vi "Main.vi"() -> ()   [LabVIEW 2013] (continued)
                n3557 = case shown="1" w6177 {
                  tunnel: w6176 -> [w6190 _]
                  frame 1 {
                    # "2nd Data Point.\nUpdate Status of c: an u: in cRIO"
                    n3558 = Index Array(array=w6190) -> (element #1=w6189:bool, element #2=w6186:bool)  [unwired: 2 in]
                    n3559 = Select(t="c: OK,", s=w6189, f="c: Fail,") -> (s? t:f=w6182:string)
                    n3560 = Select(t=" u: OK.", s=w6186, f=" u: Fail.") -> (s? t:f=w6181:string)
                    n3561 = Concatenate Strings("{Running Process} cRIO data file created status: ", w6182, w6181) -> (w6179:string)
                    n3562 = call "Queue - EnQueue to MessageQ.vi"("<NoD> Don't Display to UI"=TRUE, "Message"=w6179) -> ()  [unwired: 9 in, 1 out]
                  }
                  frame 0, Default {
                    # "Skip 1st Data Point"
                  }
                }
                n3563 = Increment(x=w6177) -> (x+1=w6178:i32)
              }
            }
          }
        }
        "Samples/ch Count" <- w5678
        n3564 = case shown="True" w5666 {
          tunnel: w5664 -> [w5698 w5745]
          tunnel: w5676 -> [w5702 w5774]
          tunnel: [w5702 w5772] -> w5675
          tunnel: [_ w5767] -> w5665
          tunnel: [w5701 w5756] -> w5673
          tunnel: w5672 -> [w5701 w5770]
          tunnel: [_ w5763] -> w5667
          tunnel: w5661 -> [_ w5750]
          frame False {
            # "t-t0"
            # "Time Not Elapse"
            n3565 = local read "Key Values"() -> (w5700:T10)
            n3566 = Bundle By Name(cluster=w5700, "Recording Duration"=w5698) -> (w5699:T10)
            n3567 = local write "Key Values"(w5699) -> ()
            n3568 = Wait Until Next ms Multiple(millisecond multiple=u32 100) -> ()  [unwired: 1 out]
            n3569 = feedback #1(0) -> (w5696:i32)
            n3570 = case shown="0" w5696 {
              frame 1, Default {
              }
              frame 0 {
                # "0 - no change"
                # "Every 10 Counts = 1sec"
                n3571 = local read "% Hold Flashing FLAG"() -> (w5707:bool)
                n3572 = Not(x=w5707) -> (.not. x?=→"% Hold Flashing FLAG":bool)
                n3573 = case shown="True" w5707 {
                  tunnel: [w5715 w5727] -> w5708
                  tunnel: 3.0 ("lower limit") -> [w5710 w5722]
                  tunnel: [u32 0 w5721] -> w5703
                  tunnel: u32 655580 -> [_ w5720]
                  frame False {
                    # "Minus When False"
                    n3574 = local read "% Hold. Time Completed"() -> (w5711:dbl)
                    n3575 = In Range and Coerce(upper limit=95.0, x=w5711, lower limit=10.0) -> (In Range?=w5712:bool)  [unwired: 1 out]
                    n3576 = case shown="False" w5712 {
                      tunnel: [w5716 w5719] -> w5715
                      tunnel: w5711 -> [w5716 w5718]
                      tunnel: w5710 -> [_ w5717]
                      frame False {
                      }
                      frame True {
                        n3577 = Subtract(x=w5718, y=w5717) -> (x-y=w5719:dbl)
                      }
                    }
                  }
                  frame True {
                    # "Add when TRUE"
                    n3578 = local read "% Hold. Time Completed"() -> (w5724:dbl)
                    n3579 = In Range and Coerce(upper limit=90.0, x=w5724, lower limit=5.0) -> (In Range?=w5723:bool)  [unwired: 1 out]
                    n3580 = case shown="True" w5723 {
                      tunnel: [w5729 w5733] -> w5727
                      tunnel: w5724 -> [w5729 w5732]
                      tunnel: w5722 -> [_ w5731]
                      tunnel: [u32 0 w5730] -> w5721
                      tunnel: w5720 -> [_ w5730]
                      frame False {
                      }
                      frame True {
                        n3581 = Add(x=w5732, y=w5731) -> (x+y=w5733:dbl)
                      }
                    }
                  }
                }
                n3582 = local write "% Hold. Time Completed"(w5708) -> ()
                n3583 = disable-structure shown="Disabled" {
                  frame Disabled {
                    # "We will not write the numerical\nindicator here :)"
                    n3584 = local read "% Hold. Time Completed (Num)"() -> ()  [unwired: 1 in]
                  }
                  frame Enabled {
                  }
                }
                n3585 = property class="DigNum (strict)"("NumText.FontColor"=w5703) -> ()  [unwired: 2 in, 2 out]
              }
            }
            n3586 = Increment(x=w5696) -> (x+1=w5694:i32)
            n3587 = Quotient & Remainder(x=w5694, y=10) -> (x-y*floor(x/y)=w5692:i32)  [unwired: 1 out]
            n3588 = feedback-in #1(w5692) -> ()
          }
          frame True {
            # "ProgStatus\n1 - Not running (Background)\n2 - RUN (Green)\n4 - RUN HLD (Red)\n8 - HLD Flashing (Red)"
            # "Segment.Type\n0 - End\n1 - Rate\n3 - Dwell"
            # "ProgStatus\n1 - Not running\n2 - RUN\n4 - RUN HLD\n8 - HLD Flashing"
            # "Time Elapsed"
            n3589 = local read "VISA resource name RS232"() -> (w5769:string)
            n3590 = local read "Simulate ET3500"() -> (w5735:bool)
            n3591 = local read "ET3500 Error"() -> (w5768:errorcluster)
            n3592 = control-ref of="ET3504 Status"() -> (w5743:refnum<vi>)
            n3593 = call "ET3500 - Read Program Parameters.vi"("Sample/ch per Count"=w5750, "Simulate"=w5735, "ET3500 Status"=w5743, "error in (no error)"=w5768, "subVI (Auto Interactive)"=TRUE ("subVI"), "Option"=cluster{"Init":bool, "Close":bool} {"Init"=FALSE, "Close"=FALSE}, "VISA resource name"=w5769) -> ("error out"=w5759:errorcluster, "Segment.Type"=w5758:i16, "Parameter Cluster (Scaled)"=w5757:T76, "Segment.Duration (min)"=w5771:dbl)  [unwired: 1 out]
            "Parameter Cluster (Scaled)" <- w5757
            n3594 = local read "TransactionRunNo (Execute)"() -> (w5752:string)
            n3595 = Unbundle By Name(w5757) -> ("SegTimeLeft (min)"=w5776:dbl, "PVIn (degC)"=w5741:dbl, "ProgStatus"=w5775:i16)
            n3596 = local read "Transaction No (Execute)"() -> (w5754:string)
            n3597 = control-ref of="WPS Details Setup"() -> (w5755:refnum<vi>)
            n3598 = control-ref of="Sequence Status"() -> (w5760:refnum<vi>)
            n3599 = control-ref of="MCListBox FHS Setup"() -> (w5761:refnum<vi>)
            n3600 = And(x=w5735, y="Simulate Hold Temp Inc") -> (x .and. y?=w5739:bool)
            n3601 = local read "DB - Active Process"() -> (w5744:bool)
            n3602 = local read "DB - Transaction"() -> (w5751:bool)
            n3603 = Bundle("Transaction No (Execute)"=w5754, "TransactionRunNo (Execute)"=w5752) -> (w5753:T77)  [unwired: 1 in]
            n3604 = Select(t="Simulate Hold Temp Inc", s=w5739, f=0.0) -> (s? t:f=w5737:dbl)
            n3605 = Select(t=errorcluster {"status"=TRUE, "code"=-1000, "source"="Simulate ET3500 Error. "} ("Error Out"), s="Simulate ET3500 Error", f=w5759) -> (s? t:f=w5763:errorcluster)
            n3606 = Add(x=w5741, y=w5737) -> (x+y=w5740:dbl)
            n3607 = call "Status - Update Sequence Status.vi"("Sequence Status"=w5760, "WPS Details"=w5755, "DB - Transaction"=w5751, "Transaction"=w5753, "MCListBox FHS Setup"=w5761, "ET3504 Status"=w5743, "Error In"=w5759, "Parameter Cluster (Scaled)"=w5757, "DB - Active Process"=w5744, "Segment.Type"=w5758) -> ("Segment.Type II"=w5756:i16, "Error Out"=→"System Status":errorcluster)  [unwired: 4 in]
            n3608 = local write "ET3500 Error"(w5763) -> ()
            n3609 = To Long Integer(number=w5775) -> (32bit integer=w5773:i32)
            n3610 = case shown="\"Running\"" w5774 {
              selector: w5774 -> [w5798 w5807 w5830]
              tunnel: w5773 -> [w5802 w5810 _]
              tunnel: [w5799 w5808 w5830] -> w5772
              tunnel: [_ _ TRUE] -> w5767
              tunnel: w5740 -> [_ w5806 _]
              frame "Wait For RUN", Default {
                n3611 = Equal?(x=w5802, y=2) -> (x = y?=w5800:bool)
                n3612 = case shown="True" w5800 {
                  tunnel: [w5803 ET3500_Program_Status."Running"] -> w5799
                  tunnel: w5798 -> [w5803 _]
                  frame False {
                  }
                  frame True {
                  }
                }
              }
              frame "Running" {
                # "Wait For Stop"
                n3613 = case shown="True" "Stop On Final Target Temperature" {
                  tunnel: w5810 -> [w5813 _]
                  tunnel: [w5811 w5824] -> w5809
                  tunnel: w5806 -> [_ w5816]
                  frame False {
                    n3614 = Equal?(x=w5813, y=1) -> (x = y?=w5811:bool)
                  }
                  frame True {
                    # "If error any of these\nwill be  ZERO.\nThis is now the ERROR\ncheck condition\nof this STATE"
                    n3615 = local read "Final Target Temperature"() -> (w5823:cluster{"Final Target Temperature":string})
                    n3616 = Unbundle By Name(w5823) -> ("Final Target Temperature"=w5822:string)
                    n3617 = local read "Hold Time Completed"() -> (w5825:bool)
                    n3618 = local read "1st TC"() -> (w5817:dbl)
                    n3619 = Decimal String To Number(string=w5822) -> (number=w5820:i32)  [unwired: 2 in, 1 out]
                    n3620 = Add(x="Final Target Temp Offset", y=w5820) -> (x+y=w5819:i32)
                    "Final Target + Offset\n(Updated Only when active)" <- w5819
                    n3621 = Less Or Equal?(x=w5817, y=w5819) -> (x <= y?=w5818:bool)
                    n3622 = Less Or Equal?(x=w5816, y=w5819) -> (x <= y?=w5826:bool)
                    n3623 = Multiply(x=w5817, y=w5816) -> (x*y=w5815:dbl)
                    n3624 = Greater Than 0?(x=w5815) -> (x > 0?=w5814:bool)
                    n3625 = Compound Arithmetic op=AND "AND"(w5814, w5818, w5826, w5825) -> (w5824:bool)
                  }
                }
                n3626 = case shown="False" w5809 {
                  tunnel: [w5827 ET3500_Program_Status."Stopped"] -> w5808
                  tunnel: w5807 -> [w5827 _]
                  frame False {
                    # "Keep Waiting"
                  }
                  frame True {
                    # "Stopped"
                  }
                }
              }
              frame "Stopped" {
              }
            }
            n3627 = case shown="3" w5756 {
              tunnel: [w5836 w5927 w6039] -> w5742
              tunnel: w5776 -> [_ w5929 _]
              tunnel: w5771 -> [_ w5938 _]
              tunnel: w5770 -> [w5832 w5941 _]
              tunnel: w5740 -> [w5831 w5931 _]
              frame 0, Default {
                # "Not Ended yet?"
                # "CURRENT STATE:   End (0) or Rate (1) or ERROR"
                n3628 = case shown="3" w5832 {
                  tunnel: w5831 -> [_ w5867]
                  frame 0, Default {
                    # "PREVIOUS STATE:   End (0) or ERROR"
                  }
                  frame 3 {
                    w5853 = 1  # Value
                    w5852 = 2  # Recorded Hold Time
                    w5865 = cluster{"Color Box":u32, "Color Box 2":u32}[] [{"Color Box"=16711680, "Color Box 2"=16711680}, {"Color Box"=6618880, "Color Box 2"=6618880}, {"Color Box"=4934475, "Color Box 2"=4934475}, {"Color Box"=6618880, "Color Box 2"=6618880}]  # False is Now RED (Prev Grey)
                    # "PREVIOUS STATE:  Dwell (3)\nSo now Main Hold (Dwell) is OVER"
                    n3629 = local read "DB - Transaction"() -> (w5862:bool)
                    n3630 = local read "Simulate cRIO"() -> (w5848:bool)
                    n3631 = local read "Simulated TimeStamp"() -> (w5849:timestamp)
                    n3632 = local read "Parameter (Start Dwell Time)"() -> (w5864:timestamp)
                    n3633 = Get Date/Time In Seconds() -> (seconds since 1Jan1904=w5861:timestamp)
                    n3634 = And(x="Simulate Hold Time Inc", y=w5848) -> (x .and. y?=w5846:bool)
                    n3635 = Select(t="Simulate Hold Time Inc (s)", s=w5846, f=0.0) -> (s? t:f=w5843:dbl)
                    n3636 = Add(x=w5849, y=w5843) -> (x+y=w5842:timestamp)
                    n3637 = Select(t=w5842, s=w5848, f=w5861) -> (s? t:f=w5860:timestamp)
                    "Parameter (End Dwell Time)" <- w5860
                    n3638 = local read "Display Start Stop Marker"() -> (w5854:bool)
                    n3639 = local read "Info."() -> (w5863:T9)
                    n3640 = call "Parameters - Update.vi"("Parameter (End Dwell Temp)"=w5867, "Parameter (End Dwell Time)"=w5860, "Parameter (Start Dwell Time)"=w5864, "Info."=w5863) -> ("Variant Allowed (Hold Time)"=w5841:bool, "Cluster"=w5866:T78, "Parameters"=w5851:string[][])  [unwired: 4 in, 1 out]
                    n3641 = property on="Variant Allowed (Hold Time)" class="Bool (strict)"("Colors [4]"=w5865, "Value"=w5841) -> ()  [unwired: 2 in, 2 out]
                    n3642 = Index Array(array=w5851, index (row)=w5852, index (col)=w5853) -> (element=w5850:string)
                    n3643 = case shown="False" w5841 {
                      tunnel: w5850 -> [w5874 w5877]
                      frame True {
                        # "Hold Duration Variant OK."
                        n3644 = Concatenate Strings("{RUNNING Process} " ("string"), "Recorded Hold Duration is " ("string"), w5874, " (HH:MM)" ("string")) -> (w5872:string)
                        n3645 = call "Queue - EnQueue to MessageQ.vi"("<NoD> Don't Display to UI"=TRUE, "Message"=w5872) -> ()  [unwired: 9 in, 1 out]
                      }
                      frame False {
                        # "Hold Duration Variant Failed!"
                        n3646 = flat-sequence {
                          tunnel: w5877 -> [w5879]
                          tunnel: ["<E 306>"] -> w5876
                          frame #0 {
                            n3647 = Format Date/Time String() -> ()  [unwired: 3 in, 1 out]
                            "<current hold time> ON Failing Hold Time Variance" <- w5879
                          }
                        }
                        n3648 = property on="Toggle ET3500 Error" class="Str"("Val(Sgnl)"=w5876) -> ()  [unwired: 2 in, 2 out]
                      }
                    }
                    n3649 = case shown="True" w5854 {
                      tunnel: w5860 -> [_ w5881]
                      frame False {
                      }
                      frame True {
                        n3650 = To Double Precision Float(number=w5881) -> (double precision float=w5883:dbl)
                        n3651 = property on="Chart" class="WFChart (strict)"() -> ("XScale.MarkerVals[]"=w5880:dbl[])  [unwired: 2 in, 2 out]
                        n3652 = Build Array (concatenate)(w5880, w5883) -> (w5882:dbl[])
                        n3653 = property on="Chart" class="WFChart (strict)"("XScale.MarkerVals[]"=w5882) -> ()  [unwired: 2 in, 2 out]
                      }
                    }
                    n3654 = Unbundle By Name(w5866) -> ("End Holding Time & Date"=w5857:string, "End Holding Temperature"=w5856:string)
                    n3655 = property on="End Holding Time and Date" class="Str"("Value"=w5857) -> (error out=w5859:errorcluster)  [unwired: 2 in, 1 out]
                    n3656 = property on="End Holding Temperature" class="Str"("Value"=w5856) -> (error out=w5858:errorcluster)  [unwired: 2 in, 1 out]
                    n3657 = case shown="True" w5841 {
                      frame False {
                      }
                      frame True {
                        n3658 = property on="% Hold. Time Completed" class="Slide (strict)"() -> ("Scale.Maximum"=w5868:dbl)  [unwired: 2 in, 2 out]
                        n3659 = local write "% Hold. Time Completed (Num)"(w5868) -> ()
                        n3660 = local write "% Hold. Time Completed"(w5868) -> ()
                        n3661 = local write "Hold Time Completed"(TRUE ("Hold Time Completed")) -> ()
                      }
                    }
                    n3662 = Merge Errors(w5859, w5858) -> (w5855:errorcluster)
                    n3663 = case shown="True" w5862 {
                      tunnel: w5851 -> [_ w5917]
                      tunnel: w5857 -> [_ w5906]
                      tunnel: w5856 -> [_ w5916]
                      tunnel: w5841 -> [_ w5897]
                      tunnel: w5855 -> [w5884 _]
                      frame False {
                        n3664 = local read "Latest stp file"() -> (w5890:path)
                        n3665 = control-ref of="Parameter Buffer"() -> (w5891:refnum<vi>)
                        n3666 = call <vilib>:"Open Config Data.vi"("error in (no error)"=w5884, "create file if necessary (T)"=FALSE, "configuration file path"=w5890) -> ("error out"=w5887:errorcluster, "refnum"=w5889:T59)  [unwired: 6 in, 1 out]
                        n3667 = call "Key - Cluster Write.vi"("error in (no error)"=w5887, "Cluster Ref in"=w5891, "Refnum in"=w5889) -> ("error out"=w5886:errorcluster, "Refnum out"=w5888:T59)  [unwired: 7 in]
                        n3668 = call <vilib>:"Close Config Data.vi"("error in (no error)"=w5886, "write file if changed (T)"=TRUE, "refnum"=w5888) -> ("error out"=w5892:errorcluster)  [unwired: 7 in, 1 out]
                        n3669 = local write "stp file Error Out"(w5892) -> ()
                      }
                      frame True {
                        w5911 = T63[] [enum."[EndHoldTime]", enum."[HoldTimePercentage]", enum."[HoldProgressColor]"] items=["[IsActive]", "[TransactionNo]", "[TransactionRunNo]", "[SequenceStatus]", "[StartRecordTime]", "[EndRecordTime]", "[StartHoldTime]", "[EndHoldTime]", "[Message1]", "[Message2]", "[HoldTimeRemaining]", "[HoldTimePercentage]", "[HoldProgressColor]", "[OrderNumbers]", "[CurrentTemp]", "[UnitOfTemperature]", "[IsAppClientLive]", "[RawDataFile]", "[RecordedMinutes]", "[FurnaceControlStatus]", "[FurnaceControlColor]", "[ControllerStatus]", "[ControllerColor]", "[IsControllerOnline]", "[ProcessColor]", "[OverallColor]", "[LastUpdatedOn]", "[LastUpdatedCmsTime]", "[Inactive]"] ("[Execute].[ActiveProcess]\n2014-10-14 14:58")
                        w5912 = 2  # Recorded Hold Time
                        w5925 = T62[] [enum."[EndHoldTime]", enum."[EndHoldTemp]", enum."[HoldDurationMinutes]", enum."[HoldTimePercentage]", enum."[IsTimeWithinTol]"] items=["[StartRecordTime]", "[StartRecordTemp]", "[MaxRecordedTemp]", "[MaxRecordedTempTime]", "[MinRecordedTemp]", "[MinRecordedTempTime]", "[EndRecordTemp]", "[EndRecordTime]", "[RecordedMinutes]", "[StartHoldTime]", "[StartHoldTemp]", "[HoldTimeMaxTemp]", "[HoldTimeMaxTempTime]", "[HoldTimeMinTemp]", "[HoldTimeMinTempTime]", "[EndHoldTime]", "[EndHoldTemp]", "[HoldDurationMinutes]", "[TempDiffDuringHold]", "[UnitOfTemperature]", "[PerformedBy]", "[PerformedOn]", "[IsTempWithinTol]", "[IsTimeWithinTol]", "[HoldTimePercentage]", "[ProcessStatus]", "[OverallStatus]", "[SequenceStatus]", "[Parameter1]", "[Parameter2]", "[Parameter3]", "[Parameter4]", "[Parameter5]", "[Parameter6]", "[Parameter7]", "[Parameter8]", "[Parameter9]", "[Parameter10]", "[Parameter11]", "[Parameter12]", "[Result]", "[RawDataFile]", "[RawDataFilePath]", "[RawDataFileName]", "[OutputSetId]", "[SavedBy]", "[SavedOn]", "[Inactive]"]  # [TransactionResult] v02
                        # "[TempDiffDuringHold] will be updated when Recipe End ONLY"
                        n3670 = local read "Hold Time %"() -> (w5895:string)
                        n3671 = Select(t="1", s=w5897, f="0") -> (s? t:f=w5910:string)
                        n3672 = Select(t="100", s=w5897, f=w5895) -> (s? t:f=w5894:string)
                        n3673 = Index Array(array=w5917, index (col)=1 ("disabled index (col)")) -> (element=w5914:string[])  [unwired: 1 in]
                        n3674 = Index Array(array=w5914, index=w5912) -> (element=w5913:string)
                        n3675 = local read "TransactionRunNo"() -> (w5919:string)
                        n3676 = local read "Transaction No"() -> (w5920:string)
                        n3677 = Bundle("Transaction No"=w5920, "TransactionRunNo"=w5919) -> (w5918:T61)  [unwired: 1 in]
                        n3678 = Build Array(w5906, w5916, w5913, w5894, w5910) -> (w5924:string[])
                        n3679 = call "DB - [Execute].[Transaction].vi"("DB.Schema.Table"="SRTRS.Execute.TransactionResult", "Transaction"=w5918, "DB - Execute Transaction"=DB_-_Execute_Transaction_Enum."UPDATE [TransactionResult]" ("DB - Setup Item Enum"), "[TransactionResult] v02"=w5925, "<Values>"=w5924) -> ("SUMMARY"=w5902:errorcluster)  [unwired: 11 in, 3 out]
                        n3680 = local write "DB"(w5902) -> ()
                        n3681 = control-ref of="Hold Time Completed"() -> (w5900:refnum<vi>)
                        n3682 = global read "Global SRTRS.vi" "Logon"() -> (w5909:T21)
                        n3683 = Unbundle By Name(w5909) -> ("PlantID"=w5908:string, "SystemID"=w5907:string)
                        n3684 = call "String - Boolean Ref Color.vi"("Bool Refnum"=w5900) -> ("Color (U32 String)"=w5899:string)  [unwired: 4 in]
                        n3685 = Bundle("PlantID"=w5908, "SystemID"=w5907) -> (w5901:cluster{"PlantID":string, "SystemID":string})  [unwired: 1 in]
                        n3686 = Build Array(w5906, w5894, w5899) -> (w5905:string[])
                        n3687 = call "DB - [CMS].[Execute].[ActiveProcess].vi"("Application"="SRTRS", "[PlantId],[SystemId]"=w5901, "DB - CMS Execute ActiveProcess"=T74."UPDATE [Execute].[ActiveProcess]" ("DB - Execute ActiveProcess"), "[Execute].[ActiveProcess]\n2014-10-14 14:58"=w5911, "<Data>"=w5905) -> ("SUMMARY"=w5903:errorcluster)  [unwired: 11 in, 3 out]
                        n3688 = local write "DB"(w5903) -> ()
                      }
                    }
                  }
                }
                n3689 = local read "Parameter (End Dwell Time)"() -> (w5835:timestamp)
                n3690 = Equal?(x=w5835, y=timestamp(3471350400 s since 1904-01-01)) -> (x = y?=w5833:bool)
                n3691 = case shown="False" w5833 {
                  tunnel: [0.0 ("(HH:mm)") w5838] -> w5836
                  frame False {
                    # "Started and Ended"
                  }
                  frame True {
                    # "Not Started Yet"
                    n3692 = local read "Info."() -> (w5840:T9)
                    n3693 = Unbundle By Name(w5840) -> ("Hold. Time (hour:minute)"=w5839:string)
                    n3694 = call "String - Format to (HH_colon_MM).vi"("xx:xx"=w5839) -> ("seconds"=w5838:dbl)  [unwired: 9 in, 1 out]
                  }
                }
              }
              frame 3 {
                # "Hold Time (seconds)"
                # "CURRENT STATE:   Dwell (3) - Main Hold"
                n3695 = Divide(x=w5929, y=w5938) -> (x/y=w5933:dbl)
                n3696 = Subtract(x=1.0, y=w5933) -> (x-y=w5932:dbl)
                n3697 = Multiply(x=100.0, y=w5932) -> (x*y=w5930:dbl)
                n3698 = case shown="3, Default" w5941 {
                  tunnel: w5931 -> [w5942 w6003]
                  tunnel: w5930 -> [w5948 _]
                  frame 3, Default {
                    # "If FALSE previously, it will remain FALSE"
                    # "PREVIOUS STATE: Dwelling OR ERROR"
                    n3699 = local read "DB - Transaction"() -> (w5952:bool)
                    n3700 = local read "Info."() -> (w5953:T9)
                    n3701 = call "Parameters - Update.vi"("Parameter (Current Dwell Temp)"=w5942, "Info."=w5953) -> ("Variant Allowed (Current Hold Temp)"=w5944:bool)  [unwired: 6 in, 3 out]
                    n3702 = property on="Variant Allowed (Hold Temp)" class="Bool (strict)"() -> ("Value"=w5945:bool)  [unwired: 2 in, 2 out]
                    n3703 = And(x=w5945, y=w5944) -> (x .and. y?=w5946:bool)
                    n3704 = Number To Decimal String(number=w5948) -> (decimal integer string=w5947:string)  [unwired: 1 in]
                    "Hold Time %" <- w5947
                    n3705 = case shown="True" w5952 {
                      tunnel: w5946 -> [_ w5981]
                      tunnel: w5947 -> [_ w5972]
                      frame False {
                      }
                      frame True {
                        w5983 = T62[] [enum."[IsTempWithinTol]", enum."[HoldTimePercentage]"] items=["[StartRecordTime]", "[StartRecordTemp]", "[MaxRecordedTemp]", "[MaxRecordedTempTime]", "[MinRecordedTemp]", "[MinRecordedTempTime]", "[EndRecordTemp]", "[EndRecordTime]", "[RecordedMinutes]", "[StartHoldTime]", "[StartHoldTemp]", "[HoldTimeMaxTemp]", "[HoldTimeMaxTempTime]", "[HoldTimeMinTemp]", "[HoldTimeMinTempTime]", "[EndHoldTime]", "[EndHoldTemp]", "[HoldDurationMinutes]", "[TempDiffDuringHold]", "[UnitOfTemperature]", "[PerformedBy]", "[PerformedOn]", "[IsTempWithinTol]", "[IsTimeWithinTol]", "[HoldTimePercentage]", "[ProcessStatus]", "[OverallStatus]", "[SequenceStatus]", "[Parameter1]", "[Parameter2]", "[Parameter3]", "[Parameter4]", "[Parameter5]", "[Parameter6]", "[Parameter7]", "[Parameter8]", "[Parameter9]", "[Parameter10]", "[Parameter11]", "[Parameter12]", "[Result]", "[RawDataFile]", "[RawDataFilePath]", "[RawDataFileName]", "[OutputSetId]", "[SavedBy]", "[SavedOn]", "[Inactive]"]  # [TransactionResult] 2014-09-28 19:20
                        # "The indicator can show 25:59:59\ni.e. more than 23:59:59"
                        n3706 = Select(t="1", s=w5981, f="0") -> (s? t:f=w5978:string)
                        n3707 = local read "TransactionRunNo"() -> (w5975:string)
                        n3708 = Build Array(w5978, w5972) -> (w5982:string[])
                        n3709 = local read "Transaction No"() -> (w5976:string)
                        n3710 = Bundle("Transaction No"=w5976, "TransactionRunNo"=w5975) -> (w5974:T61)  [unwired: 1 in]
                        n3711 = call "DB - [Execute].[Transaction].vi"("DB.Schema.Table"="SRTRS.Execute.TransactionResult", "Transaction"=w5974, "DB - Execute Transaction"=DB_-_Execute_Transaction_Enum."UPDATE [TransactionResult]" ("DB - Setup Item Enum"), "[TransactionResult] v02"=w5983, "<Values>"=w5982) -> ("SUMMARY"=w5973:errorcluster)  [unwired: 11 in, 3 out]
                        n3712 = local write "DB"(w5973) -> ()
                      }
                    }
                    n3713 = Compound Arithmetic op=AND(w5945, invert w5944) -> (w5943:bool)
                    n3714 = property on="Variant Allowed (Hold Temp)" class="Bool (strict)"("Value"=w5946) -> ()  [unwired: 2 in, 2 out]
                    n3715 = case shown="True" w5943 {
                      tunnel: w5942 -> [_ w5955]
                      frame False {
                      }
                      frame True {
                        # "1st Time Variant Failed!"
                        n3716 = flat-sequence {
                          tunnel: w5955 -> [w5959]
                          tunnel: ["<E 305>" ("Value (Signaling)")] -> w5954
                          frame #0 {
                            n3717 = Number To Fractional String(number=w5959, precision (6)=i16 0) -> (F-format string=→"<current temperature> ON Failing Hold Temp Variance":string)  [unwired: 2 in]
                          }
                        }
                        n3718 = property on="Toggle ET3500 Error" class="Str"("Val(Sgnl)"=w5954) -> ()  [unwired: 2 in, 2 out]
                      }
                    }
                    n3719 = local read "Enable Central Monitoring"() -> (w5950:bool)
                    n3720 = local read "DB - Active Process"() -> (w5951:bool)
                    n3721 = And(x=w5950, y=w5951) -> (x .and. y?=w5949:bool)
                    n3722 = case shown="True" w5949 {
                      tunnel: w5947 -> [_ w5964]
                      frame False {
                      }
                      frame True {
                        w5967 = T63[] [enum."[HoldTimePercentage]", enum."[HoldProgressColor]"] items=["[IsActive]", "[TransactionNo]", "[TransactionRunNo]", "[SequenceStatus]", "[StartRecordTime]", "[EndRecordTime]", "[StartHoldTime]", "[EndHoldTime]", "[Message1]", "[Message2]", "[HoldTimeRemaining]", "[HoldTimePercentage]", "[HoldProgressColor]", "[OrderNumbers]", "[CurrentTemp]", "[UnitOfTemperature]", "[IsAppClientLive]", "[RawDataFile]", "[RecordedMinutes]", "[FurnaceControlStatus]", "[FurnaceControlColor]", "[ControllerStatus]", "[ControllerColor]", "[IsControllerOnline]", "[ProcessColor]", "[OverallColor]", "[LastUpdatedOn]", "[LastUpdatedCmsTime]", "[Inactive]"] ("[Execute].[ActiveProcess]\n2014-10-14 14:58")
                        n3723 = global read "Global SRTRS.vi" "Logon"() -> (w5970:T21)
                        n3724 = control-ref of="Hold Time Completed"() -> (w5962:refnum<vi>)
                        n3725 = Unbundle By Name(w5970) -> ("PlantID"=w5969:string, "SystemID"=w5968:string)
                        n3726 = call "String - Boolean Ref Color.vi"("Bool Refnum"=w5962) -> ("Color (U32 String)"=w5961:string)  [unwired: 4 in]
                        n3727 = Bundle("PlantID"=w5969, "SystemID"=w5968) -> (w5963:cluster{"PlantID":string, "SystemID":string})  [unwired: 1 in]
                        n3728 = Build Array(w5964, w5961) -> (w5966:string[])
                        n3729 = call "DB - [CMS].[Execute].[ActiveProcess].vi"("Application"="SRTRS", "[PlantId],[SystemId]"=w5963, "DB - CMS Execute ActiveProcess"=T74."UPDATE [Execute].[ActiveProcess]" ("DB - Execute ActiveProcess"), "[Execute].[ActiveProcess]\n2014-10-14 14:58"=w5967, "<Data>"=w5966) -> ("SUMMARY"=w5965:errorcluster)  [unwired: 11 in, 3 out]
                        n3730 = local write "DB"(w5965) -> ()
                      }
                    }
                  }
                  frame 1, 300 {
                    w6001 = cluster{"Color Box":u32, "Color Box 2":u32}[] [{"Color Box"=16711680, "Color Box 2"=16711680}, {"Color Box"=6618880, "Color Box 2"=6618880}, {"Color Box"=4934475, "Color Box 2"=4934475}, {"Color Box"=6618880, "Color Box 2"=6618880}]  # False is Now RED, (Prev  Grey)
                    w5991 = cluster{"Color Box":u32, "Color Box 2":u32}[] [{"Color Box"=16383786, "Color Box 2"=16383786}, {"Color Box"=6618880, "Color Box 2"=6618880}, {"Color Box"=4934475, "Color Box 2"=4934475}, {"Color Box"=6618880, "Color Box 2"=6618880}]  # False is Now Yellow (Prev Grey)
                    # "Create Start Hold Marker"
                    # "Fix ERROR here"
                    # "Initialized to TRUE"
                    # "PREVIOUS STATE:  Rate (1) or Dwell (300) => Just Entering Dwell (3)"
                    n3731 = local read "DB - Transaction"() -> (w5999:bool)
                    n3732 = local read "Simulated TimeStamp"() -> (w5998:timestamp)
                    n3733 = local read "Simulate cRIO"() -> (w5996:bool)
                    n3734 = Get Date/Time In Seconds() -> (seconds since 1Jan1904=w5997:timestamp)
                    n3735 = Select(t=w5998, s=w5996, f=w5997) -> (s? t:f=w5995:timestamp)
                    "Parameter (Start Dwell Time)" <- w5995
                    n3736 = local read "Display Start Stop Marker"() -> (w5985:bool)
                    n3737 = call "Parameters - Update.vi"("Parameter (Start Dwell Temp)"=w6003, "Parameter (Start Dwell Time)"=w5995) -> ("Cluster"=w6002:T78)  [unwired: 6 in, 3 out]
                    n3738 = Unbundle By Name(w6002) -> ("Start Holding Time & Date"=w5988:string, "Start Holding Temperature"=w5987:string)
                    n3739 = property on="Start Holding Temperature" class="Str"("Value"=w5987) -> (error out=w5989:errorcluster)  [unwired: 2 in, 1 out]
                    n3740 = property on="Start Holding Time and Date" class="Str"("Value"=w5988) -> (error out=w5990:errorcluster)  [unwired: 2 in, 1 out]
                    n3741 = local read "Enable Central Monitoring"() -> (w5993:bool)
                    n3742 = local read "DB - Active Process"() -> (w5994:bool)
                    n3743 = case shown="True" w5985 {
                      tunnel: w5995 -> [_ w6004]
                      frame False {
                      }
                      frame True {
                        n3744 = To Double Precision Float(number=w6004) -> (double precision float=w6006:dbl)
                        n3745 = Build Array(w6006) -> (w6005:dbl[])
                        n3746 = property on="Chart" class="WFChart (strict)"("XScale.MarkerVals[]"=w6005) -> ()  [unwired: 2 in, 2 out]
                      }
                    }
                    n3747 = Merge Errors(w5990, w5989) -> (w5986:errorcluster)
                    n3748 = case shown="True" w5999 {
                      tunnel: w5988 -> [_ w6030]
                      tunnel: w5987 -> [_ w6035]
                      tunnel: w5986 -> [w6020 _]
                      frame False {
                        n3749 = local read "Latest stp file"() -> (w6026:path)
                        n3750 = control-ref of="Parameter Buffer"() -> (w6027:refnum<vi>)
                        n3751 = call <vilib>:"Open Config Data.vi"("error in (no error)"=w6020, "create file if necessary (T)"=FALSE, "configuration file path"=w6026) -> ("error out"=w6023:errorcluster, "refnum"=w6025:T59)  [unwired: 6 in, 1 out]
                        n3752 = call "Key - Cluster Write.vi"("error in (no error)"=w6023, "Cluster Ref in"=w6027, "Refnum in"=w6025) -> ("error out"=w6022:errorcluster, "Refnum out"=w6024:T59)  [unwired: 7 in]
                        n3753 = call <vilib>:"Close Config Data.vi"("error in (no error)"=w6022, "refnum"=w6024) -> ("error out"=→"stp file Error Out":errorcluster)  [unwired: 8 in, 1 out]
                      }
                      frame True {
                        w6036 = T62[] [enum."[StartHoldTime]", enum."[StartHoldTemp]"] items=["[StartRecordTime]", "[StartRecordTemp]", "[MaxRecordedTemp]", "[MaxRecordedTempTime]", "[MinRecordedTemp]", "[MinRecordedTempTime]", "[EndRecordTemp]", "[EndRecordTime]", "[RecordedMinutes]", "[StartHoldTime]", "[StartHoldTemp]", "[HoldTimeMaxTemp]", "[HoldTimeMaxTempTime]", "[HoldTimeMinTemp]", "[HoldTimeMinTempTime]", "[EndHoldTime]", "[EndHoldTemp]", "[HoldDurationMinutes]", "[TempDiffDuringHold]", "[UnitOfTemperature]", "[PerformedBy]", "[PerformedOn]", "[IsTempWithinTol]", "[IsTimeWithinTol]", "[HoldTimePercentage]", "[ProcessStatus]", "[OverallStatus]", "[SequenceStatus]", "[Parameter1]", "[Parameter2]", "[Parameter3]", "[Parameter4]", "[Parameter5]", "[Parameter6]", "[Parameter7]", "[Parameter8]", "[Parameter9]", "[Parameter10]", "[Parameter11]", "[Parameter12]", "[Result]", "[RawDataFile]", "[RawDataFilePath]", "[RawDataFileName]", "[OutputSetId]", "[SavedBy]", "[SavedOn]", "[Inactive]"]  # [TransactionResult] 2014-09-28 19:20
                        n3754 = local read "TransactionRunNo"() -> (w6032:string)
                        n3755 = Build Array(w6030, w6035) -> (w6031:string[])
                        n3756 = local read "Transaction No"() -> (w6033:string)
                        n3757 = Bundle("Transaction No"=w6033, "TransactionRunNo"=w6032) -> (w6034:T61)  [unwired: 1 in]
                        n3758 = call "DB - [Execute].[Transaction].vi"("DB.Schema.Table"="SRTRS.Execute.TransactionResult", "Transaction"=w6034, "DB - Execute Transaction"=DB_-_Execute_Transaction_Enum."UPDATE [TransactionResult]" ("DB - Setup Item Enum"), "[TransactionResult] v02"=w6036, "<Values>"=w6031) -> ("SUMMARY"=w6029:errorcluster)  [unwired: 11 in, 3 out]
                        n3759 = local write "DB"(w6029) -> ()
                      }
                    }
                    n3760 = property on="Hold Time Completed" class="Bool (strict)"("Colors [4]"=w5991) -> ()  [unwired: 2 in, 2 out]
                    n3761 = And(x=w5993, y=w5994) -> (x .and. y?=w5992:bool)
                    n3762 = case shown="True" w5992 {
                      tunnel: w5988 -> [_ w6013]
                      tunnel: w5991 -> [_ _]
                      tunnel: w5986 -> [_ w6008]
                      frame False {
                      }
                      frame True {
                        w6015 = T63[] [enum."[StartHoldTime]", enum."[HoldProgressColor]"] items=["[IsActive]", "[TransactionNo]", "[TransactionRunNo]", "[SequenceStatus]", "[StartRecordTime]", "[EndRecordTime]", "[StartHoldTime]", "[EndHoldTime]", "[Message1]", "[Message2]", "[HoldTimeRemaining]", "[HoldTimePercentage]", "[HoldProgressColor]", "[OrderNumbers]", "[CurrentTemp]", "[UnitOfTemperature]", "[IsAppClientLive]", "[RawDataFile]", "[RecordedMinutes]", "[FurnaceControlStatus]", "[FurnaceControlColor]", "[ControllerStatus]", "[ControllerColor]", "[IsControllerOnline]", "[ProcessColor]", "[OverallColor]", "[LastUpdatedOn]", "[LastUpdatedCmsTime]", "[Inactive]"] ("[Execute].[ActiveProcess]\n2014-10-14 14:58")
                        n3763 = control-ref of="Hold Time Completed"() -> (w6010:refnum<vi>)
                        n3764 = global read "Global SRTRS.vi" "Logon"() -> (w6018:T21)
                        n3765 = call "String - Boolean Ref Color.vi"("Bool Refnum"=w6010) -> ("Color (U32 String)"=w6009:string)  [unwired: 4 in]
                        n3766 = Unbundle By Name(w6018) -> ("PlantID"=w6017:string, "SystemID"=w6016:string)
                        n3767 = Bundle("PlantID"=w6017, "SystemID"=w6016) -> (w6011:cluster{"PlantID":string, "SystemID":string})  [unwired: 1 in]
                        n3768 = Build Array(w6013, w6009) -> (w6014:string[])
                        n3769 = call "DB - [CMS].[Execute].[ActiveProcess].vi"("Application"="SRTRS", "[PlantId],[SystemId]"=w6011, "error in (no error)"=w6008, "DB - CMS Execute ActiveProcess"=T74."UPDATE [Execute].[ActiveProcess]" ("DB - Execute ActiveProcess"), "[Execute].[ActiveProcess]\n2014-10-14 14:58"=w6015, "<Data>"=w6014) -> ("SUMMARY"=w6012:errorcluster)  [unwired: 10 in, 3 out]
                        n3770 = local write "DB"(w6012) -> ()
                      }
                    }
                    n3771 = property on="Variant Allowed (Hold Temp)" class="Bool (strict)"("Colors [4]"=w6001, "Value"=TRUE) -> ()  [unwired: 2 in, 2 out]
                  }
                }
                n3772 = Greater?(x=w5930, y=99.0) -> (0:w5935:bool)
                n3773 = local write "% Hold. Time Completed"(w5930) -> ()
                n3774 = local write "% Hold. Time Completed (Num)"(w5930) -> ()
                n3775 = local write "Hold Time Completed"(w5935) -> ()
                n3776 = property on="% Hold. Time Completed" class="Slide (strict)"("Scale.Maximum"=100, "Fill Color"=u32 786176) -> ()  [unwired: 2 in, 2 out]
                n3777 = Multiply(x=w5929, y=60.0) -> (x*y=w5927:dbl)
              }
              frame 300 {
                # "No Change"
                # "CURRENT STATE:   Dwell (300) - Mini Hold"
                n3778 = local read "Key Values"() -> (w6040:T10)
                n3779 = Unbundle By Name(w6040) -> ("Remaining Hold Time"=w6039:dbl)
              }
            }
            n3780 = local write "Process Completed"(w5767) -> ()
            n3781 = local read "Enable Central Monitoring"() -> (w5748:bool)
            n3782 = local read "DB - Active Process"() -> (w5747:bool)
            n3783 = And(x=w5748, y=w5747) -> (x .and. y?=w5746:bool)
            n3784 = case shown="True" w5746 {
              tunnel: w5745 -> [_ w5783]
              tunnel: w5740 -> [_ w5785]
              tunnel: w5742 -> [_ w5782]
              frame False {
              }
              frame True {
                w5780 = 60.0  # 60sec
                w5794 = T63[] [enum."[RecordedMinutes]", enum."[HoldTimeRemaining]", enum."[CurrentTemp]"] items=["[IsActive]", "[TransactionNo]", "[TransactionRunNo]", "[SequenceStatus]", "[StartRecordTime]", "[EndRecordTime]", "[StartHoldTime]", "[EndHoldTime]", "[Message1]", "[Message2]", "[HoldTimeRemaining]", "[HoldTimePercentage]", "[HoldProgressColor]", "[OrderNumbers]", "[CurrentTemp]", "[UnitOfTemperature]", "[IsAppClientLive]", "[RawDataFile]", "[RecordedMinutes]", "[FurnaceControlStatus]", "[FurnaceControlColor]", "[ControllerStatus]", "[ControllerColor]", "[IsControllerOnline]", "[ProcessColor]", "[OverallColor]", "[LastUpdatedOn]", "[LastUpdatedCmsTime]", "[Inactive]"] ("[Execute].[ActiveProcess]\n2014-10-14 14:58")
                n3785 = global read "Global SRTRS.vi" "Logon"() -> (w5795:T21)
                n3786 = Divide(x=w5783, y=w5780) -> (x/y=w5793:dbl)
                n3787 = Divide(x=w5782, y=w5780) -> (x/y=w5781:dbl)
                n3788 = Number To Decimal String(number=w5793) -> (decimal integer string=w5792:string)  [unwired: 1 in]
                n3789 = Unbundle By Name(w5795) -> ("PlantID"=w5796:string, "SystemID"=w5797:string)
                n3790 = Number To Decimal String(number=w5781) -> (decimal integer string=w5784:string)  [unwired: 1 in]
                n3791 = Format Value(format string="%#_4", value (0)=w5785) -> (output string=w5786:string)  [unwired: 1 in]
                n3792 = Bundle("PlantID"=w5796, "SystemID"=w5797) -> (w5787:cluster{"PlantID":string, "SystemID":string})  [unwired: 1 in]
                n3793 = Build Array(w5792, w5784, w5786) -> (w5791:string[])
                n3794 = call "DB - [CMS].[Execute].[ActiveProcess].vi"("Application"="SRTRS", "[PlantId],[SystemId]"=w5787, "DB - CMS Execute ActiveProcess"=T74."UPDATE [Execute].[ActiveProcess]" ("DB - Execute ActiveProcess"), "[Execute].[ActiveProcess]\n2014-10-14 14:58"=w5794, "<Data>"=w5791) -> ("SUMMARY"=w5788:errorcluster)  [unwired: 11 in, 3 out]
                n3795 = local write "DB"(w5788) -> ()
              }
            }
            n3796 = local read "Key Values"() -> (w5766:T10)
            n3797 = Bundle By Name(cluster=w5766, "Recording Duration"=w5745, "Remaining Hold Time"=w5742, "Current Temp"=w5740) -> (w5762:T10)
            n3798 = local write "Key Values"(w5762) -> ()
          }
        }
        n3799 = case shown="True" w5665 {
          tunnel: [w6194 Enum_-_SRTRS_State."END Process" ("Enum")] -> w5685
          tunnel: w5684 -> [w6194 _]
          frame False {
            # "Keep Checking"
            n3800 = Wait Until Next ms Multiple(millisecond multiple=u32 10) -> ()  [unwired: 1 out]
          }
          frame True {
            # "Goto Next Process"
          }
        }
        n3801 = Merge Errors(w5671, w5669, w5667) -> (w5670:errorcluster)
      }
      frame "END Process" {
        # "Close ET3500"
        # "Sample/ch Count Resets"
        # "Currently no Process 2"
        # "End Monitoring ET"
        n3802 = flat-sequence {
          tunnel: w6202 -> [_]
          frame #0 {
            # "Shows on UI:\n\"Applicatoin Logging Ended.\"  /* The rest are commented out  */"
            # "Last Temp Recorded b4 ET Comm is stopped"
            # "EnQ MessageQ"
            n3803 = local read "Key Values"() -> (w6233:T10)
            n3804 = local read "Final Target + Offset\n(Updated Only when active)"() -> (w6221:i32)
            n3805 = Unbundle By Name(w6233) -> ("Current Temp"=w6232:dbl)
            n3806 = local read "1st TC"() -> (w6225:dbl)
            n3807 = Number To Fractional String(number=w6232, precision (6)=i16 1) -> (F-format string=w6230:string)  [unwired: 2 in]
            n3808 = local read "Sequence Status"() -> (w6217:string)
            n3809 = local read "ET3504 Status"() -> (w6228:string)
            n3810 = local read "cRIO Status"() -> (w6226:string)
            n3811 = Number To Fractional String(number=w6221, precision (6)=i16 1) -> (F-format string=w6220:string)  [unwired: 2 in]
            n3812 = Number To Fractional String(number=w6225, precision (6)=i16 1) -> (F-format string=w6223:string)  [unwired: 2 in]
            n3813 = Concatenate Strings(" {END Process} " ("string"), "1st TC = ", w6223, ". PVin = ", w6230, ". Final Target =  " ("string"), w6220, ". Seq Status: " ("string"), w6217, ". ET Status: " ("string"), w6228, ". cRIO Status: " ("string"), w6226) -> (w6214:string)
            n3814 = call "Queue - EnQueue to MessageQ.vi"("<NoD> Don't Display to UI"=TRUE, "Message"=w6214) -> ()  [unwired: 9 in, 1 out]
          }
        }
        n3815 = local read "Simulate ET3500"() -> (w6209:bool)
        n3816 = local read "VISA resource name RS232"() -> (w6211:string)
        n3817 = control-ref of="ET3504 Status"() -> (w6197:refnum<vi>)
        n3818 = call "ET3500 - Read Program Parameters.vi"("Simulate"=w6209, "ET3500 Status"=w6197, "subVI (Auto Interactive)"=TRUE ("subVI"), "Option"=cluster{"Init":bool, "Close":bool} {"Init"=FALSE, "Close"=TRUE}, "VISA resource name"=w6211) -> ("error out"=w6205:errorcluster, "Segment.Type"=w6204:i16, "Parameter Cluster (Scaled)"=w6203:T76)  [unwired: 2 in, 2 out]
        n3819 = local write "Parameter Cluster (Scaled)"(w6203) -> ()
        n3820 = local read "TransactionRunNo"() -> (w6200:string)
        n3821 = control-ref of="Sequence Status"() -> (w6206:refnum<vi>)
        n3822 = control-ref of="MCListBox FHS Setup"() -> (w6207:refnum<vi>)
        n3823 = local read "Transaction No"() -> (w6201:string)
        n3824 = local write "ET3500 Error"(w6205) -> ()
        n3825 = local read "DB - Active Process"() -> (w6196:bool)
        n3826 = local read "DB - Transaction"() -> (w6199:bool)
        n3827 = Bundle("Transaction No"=w6201, "TransactionRunNo"=w6200) -> (w6198:T61)  [unwired: 1 in]
        n3828 = call "Status - Update Sequence Status.vi"("Sequence Status"=w6206, "DB - Transaction"=w6199, "Transaction"=w6198, "MCListBox FHS Setup"=w6207, "ET3504 Status"=w6197, "Error In"=w6205, "Parameter Cluster (Scaled)"=w6203, "DB - Active Process"=w6196, "Segment.Type"=w6204) -> ("Error Out"=w6202:errorcluster)  [unwired: 5 in, 1 out]
      }
      frame "Spare Enum" {
        # "No need for Samples/ch Count"
        # "Nothing here"
      }
      frame "END Recipe" {
        # "END DAQ"
        # "End DAQ, Check DAQ Stop, Set Overall Status\nFTP data File from cRIO and Replace Data_Host.\nAlso copy same file to Server \nReload Chart Using cRIO's file. Copy cRIO file to Server. Update [Execute].[TransactionResult]. Report Generation (Val(Sgnl)). Update [Execute].[ActiveProcess]\nSets Report Generate (ValSgnl) to Toggle Report Generate"
        n3829 = flat-sequence {
          tunnel: [w6288] -> w6241
          tunnel: [w6287] -> w6240
          tunnel: w6238 -> [_]
          frame #0 {
            w6286 = T35 [enum."Page Enabled", enum."Page Enabled", enum."Page Enabled", enum."Page Enabled", enum."Page Enabled"] items=["Page Enabled", "Page Disabled", "Page Disabled & Grayed"]
            n3830 = property on="Tab Body" class="TabCtl (strict)"() -> ("Pages"=w6285:refnum<vi>[])  [unwired: 2 in, 2 out]
            n3831 = for {
              tunnel: w6285 -> [w6295] mode=indexing
              tunnel: w6286 -> [w6294] mode=indexing
              n3832 = property class="Page"(reference=w6295, "PageEnb"=w6294) -> ()  [unwired: 1 in, 2 out]
            }
            n3833 = disable-structure shown="Disabled" {
              frame Disabled {
                # "If TRUE use DB instead of Memory \nfor Variants Allowed"
                n3834 = local read "RecoveryFlag"() -> ()  [unwired: 1 out]
              }
              frame Enabled {
              }
            }
            n3835 = property on="Recipe Stop" class="Bool"("DisabledEnum"=T30."Disabled and Grayed Out" ("Disabled")) -> ()  [unwired: 2 in, 2 out]
            n3836 = property on="Variant Allowed (Hold Temp)" class="Bool (strict)"() -> ("Value"=w6290:bool)  [unwired: 2 in, 2 out]
            n3837 = property on="Variant Allowed (Hold Time)" class="Bool (strict)"() -> ("Value"=w6291:bool)  [unwired: 2 in, 2 out]
            n3838 = local write "Recipe Stop Flag"(FALSE ("Recipe Stop Flag")) -> ()
            n3839 = And(x=w6290, y=w6291) -> (x .and. y?=w6287:bool)
            n3840 = property on="Overall Status" class="Bool (strict)"("Colors [4]"=cluster{"Color Box":u32, "Color Box 2":u32}[] [{"Color Box"=16727850, "Color Box 2"=16711680}, {"Color Box"=6618880, "Color Box 2"=6618880}, {"Color Box"=4934475, "Color Box 2"=4934475}, {"Color Box"=6618880, "Color Box 2"=6618880}] ("Init"), "Value"=w6287) -> (error out=w6288:errorcluster)  [unwired: 2 in, 1 out]
          }
        }
        n3841 = local read "Logged File Ref"() -> (w6266:refnum<file>)
        n3842 = flat-sequence {
          tunnel: [w6269] -> w6238
          frame #0 {
            n3843 = disable-structure shown="Disabled" {
              frame Disabled {
                n3844 = local read "Process Completed"() -> ()  [unwired: 1 out]
              }
              frame Enabled {
              }
            }
            n3845 = local read "TransactionRunNo (Execute)"() -> (w6272:string)
            n3846 = local read "Transaction No (Execute)"() -> (w6274:string)
            n3847 = local read "Manual Stop"() -> (w6270:bool)
            n3848 = case shown="True" w6270 {
              tunnel: ["<I 310>" ("<.?....> Message Code") "<I 309>" ("<.?....> Message Code")] -> w6277
              tunnel: [" process completed sucessfully." ("Description (When DB Not Available)") " process stopped" ("Description (When DB Not Available)")] -> w6276
              tunnel: ["Process Completed" ("Description (When DB Not Available)") "Process Stopped" ("Description (When DB Not Available)")] -> w6275
              frame False {
                # "Process Completed Normally"
              }
              frame True {
                # "Manual Stop is TRUE"
                n3849 = local write "Manual Stop"(FALSE ("Manual Stop")) -> ()
              }
            }
            n3850 = Concatenate Strings(w6274, ", " ("string"), w6272) -> (w6271:string)
            n3851 = call "Msgbox - Message Handler.vi"("Short Description (When DB Not Available)"=w6275, "Description (When DB Not Available)"=w6276, "Pre-Description"=w6271, "<.?....> Message Code"=w6277) -> ("MHandler Error"=w6269:errorcluster)  [unwired: 5 in, 2 out]
            n3852 = local write "MHandler"(w6269) -> ()
          }
        }
        n3853 = local read "Simulate cRIO"() -> (w6252:bool)
        n3854 = Close File(refnum=w6266) -> (error out=w6259:errorcluster)  [unwired: 1 in, 1 out]
        n3855 = local read "cRIO shared variable RT Library"() -> (w6256:string)
        n3856 = control-ref of="cRIO Status"() -> (w6247:refnum<vi>)
        n3857 = flat-sequence {
          tunnel: w6259 -> [_]
          tunnel: w6250 -> [w6531]
          tunnel: w6254 -> [w6533]
          tunnel: w6253 -> [w6532]
          frame #0 {
            # "Get YYYY\\MM from cRIO data file"
            # "Server"
            # "Create Server Data Folder if not exsits.\nCopy raw data file (either FTP-ed version from cRIO OR original Data_Host (if FTP Failed) to Server."
            n3858 = Strip Path(path=w6533) -> (stripped path=w6547:path, name=w6536:string)
            n3859 = Strip Path "Month"(path=w6547) -> (stripped path=w6546:path, name=w6544:string)
            n3860 = Strip Path "Year"(path=w6546) -> (name=w6545:string)  [unwired: 1 out]
            n3861 = local read "Data"() -> (w6543:path)
            n3862 = Concatenate Strings(w6545, "\\" ("string"), w6544) -> (w6542:string)
            n3863 = Build Path(base path=w6543, name or relative path=w6542) -> (appended path=w6537:path)
            n3864 = Build Path(base path=w6537, name or relative path=w6536) -> (appended path=w6527:path)
            n3865 = call <vilib>:"Check if File or Folder Exists.vi"("path"=w6537) -> ("error out"=w6538:errorcluster, "file or folder exists?"=w6540:bool, "dup path"=w6539:path)  [unwired: 8 in]
            n3866 = case shown="False" w6540 {
              tunnel: w6539 -> [w6557 w6559]
              tunnel: [w6556 w6559] -> _
              tunnel: [w6555 w6558] -> w6535
              tunnel: w6538 -> [w6554 w6558]
              frame False {
                # "Create Folder if NOT found\nCreate NEW"
                n3867 = Create Folder(path (use dialog)=w6557, error in=w6554) -> (created path=w6556:path, error out=w6555:errorcluster)  [unwired: 1 in, 1 out]
              }
              frame True {
                # "Folder Found"
              }
            }
            n3868 = Copy(8:w6535, 10:w6527, 11:w6531) -> (0:w6534:errorcluster)  [unwired: 2 in, 2 out]
            n3869 = local write "Data File Error"(w6534) -> ()
            n3870 = Path To String(path=w6527) -> (string=w6530:string)
            n3871 = Concatenate Strings(" File: \"" ("string"), w6530, "\"" ("string")) -> (w6526:string)
            n3872 = case shown="Error" w6534 {
              tunnel: w6532 -> [_ _]
              tunnel: w6531 -> [_ _]
              tunnel: w6527 -> [_ _]
              tunnel: w6526 -> [w6549 w6552]
              tunnel: [w6548 w6551] -> w6523
              frame No Error {
                n3873 = Concatenate Strings("File copy to Server OK." ("message"), w6549) -> (w6548:string)
              }
              frame Error {
                n3874 = Concatenate Strings("File copy to Server failed." ("message"), w6552) -> (w6551:string)
              }
            }
            n3875 = Concatenate Strings("{END Recipe} " ("string"), w6523) -> (w6522:string)
            n3876 = call "Queue - EnQueue to MessageQ.vi"("<NoD> Don't Display to UI"=TRUE, "Message"=w6522) -> ()  [unwired: 9 in, 1 out]
          }
        }
        n3877 = call "cRIO - Shared Variable RW.vi"("shared variable RT Library"=w6256, "Read/Write"=cRIO_RW_Enum."Read", "cRIO Status"=w6247) -> ("Data Path Name"=w6255:string, "Error Out"=w6258:errorcluster)  [unwired: 8 in, 7 out]
        "Data Path Name (cRIO SV)" <- w6255
        n3878 = case shown="False" w6252 {
          tunnel: w6255 -> [w6503 _]
          tunnel: [w6494 w6519] -> w6250
          tunnel: [w6501 w6519] -> w6254
          tunnel: [w6499 errorcluster {"status"=FALSE, "code"=0, "source"="FTP Skipped"} ("error out")] -> w6249
          frame False {
            w6496 = "\"" ("string")
            # "Change \n/c/ni-rt/LabVIEW Data/SRTRS4070/Data/2014/08/0090300742_20140822_114859.dat\nTO\nc:\\ni-rt\\LabVIEW Data\\SRTRS4070\\Data\\2014\\04\\0090300742_20140822_114859.dat"
            # "Auto FTP Raw Data File  from cRIO AND Replaces data file in Data_Host\nSimilar Step as {START Recovery}"
            n3879 = Search and Replace String(replace all?=TRUE ("replace all? (F)"), input string=w6503, search string="/", replace string="\\" ("replace string (\"\")")) -> (result string=w6506:string)  [unwired: 4 in, 3 out]
            n3880 = Search and Replace String(input string=w6506, search string="\\c", replace string="c:" ("replace string (\"\")")) -> (result string=w6495:string)  [unwired: 5 in, 3 out]
            n3881 = String To Path(string=w6495) -> (path=w6501:path)
            n3882 = Strip Path "<>.dat"(path=w6501) -> (name=w6502:string)  [unwired: 1 out]
            n3883 = local read "Data_Host"() -> (w6500:path)
            n3884 = Build Path(base path=w6500, name or relative path=w6502) -> (appended path=w6494:path)
            n3885 = local read "cRIO IP"() -> (w6510:string)
            n3886 = Path To String(path=w6494) -> (string=w6493:string)
            n3887 = call <vilib>:"FTP Get File.vi"("password"="", "user"="anonymous", "local path"=w6494, "remote path"=w6495, "host"=w6510) -> ("error out"=w6499:errorcluster)  [unwired: 5 in, 1 out]
            n3888 = case shown="Error" w6499 {
              tunnel: ["{END Recipe} FTP OK. " "{END Recipe} FTP failed. "] -> w6491
              frame No Error {
              }
              frame Error {
                n3889 = call "Msgbox - Message Handler.vi"("Short Description (When DB Not Available)"="FTP Error", "Description (When DB Not Available)"="Cannot FTP from cRIO.", "<.?....> Message Code"="<E 408>") -> ("MHandler Error"=w6517:errorcluster)  [unwired: 6 in, 2 out]
                n3890 = local write "MHandler"(w6517) -> ()
              }
            }
            n3891 = Concatenate Strings(w6491, "cRIO File: " ("string"), w6496, w6495, w6496, " Host File: " ("string"), w6496, w6493, w6496) -> (w6490:string)
            n3892 = call "Queue - EnQueue to MessageQ.vi"("<NoD> Don't Display to UI"=TRUE, "Message"=w6490) -> ()  [unwired: 9 in, 1 out]
          }
          frame True {
            (unwired) "FTP skipped. "
            # "c:\\temp\\SRTRS4070_Host\\Data_Host\\2014\\08\\0090300742_20140822_114859.dat"
            # "Skip FTP in Simulate cRIO Mode\nRaw Data file is using the original data file in Data_Host"
            n3893 = local read "Raw Data File"() -> (w6520:string)
            n3894 = String To Path(string=w6520) -> (path=w6519:path)
          }
        }
        n3895 = flat-sequence {
          frame #0 {
            # "Clears Raw Data File entry in ini"
